vi "Create Map from Messages to Value Indexes.vi"(8 "error in":errorcluster, 9 "module reference":T3, 10 "1553 channel handles":T4[](array[typedef]) {"terminal status channels" format="%.0x"; "error count channel refs"."wrong sync" format="%.0x"; "error count channel refs"."word" format="%.0x"; "error count channel refs"."unconfigured frames" format="%.0x"; "error count channel refs"."parity" format="%.0x"; "error count channel refs"."monitor" format="%.0x"; "error count channel refs"."Manchester" format="%.0x"; "error count channel refs"."improper number of words" format="%.0x"; "error count channel refs"."general protocol" format="%.0x"; "messages"."Rx status handles" format="%.0x"; "messages"."Tx status handles" format="%.0x"; "messages"."timestamps" format="%.0x"; "messages"."parameters"."RxBC channel handle" format="%.0x"; "messages"."parameters"."RxRT channel handle" format="%.0x"; "messages"."parameters"."Tx channel handle" format="%.0x"}, 11 "1553 channels":T9[](array[typedef])) -> (0 "error out":errorcluster, 1 "Rx read info":T1[](array[typedef]), 2 "status lookup data":T2[](array[typedef]) {"terminal address" format="%.0x"; "remote terminal handle" format="%.0x"}, 3 "map from messages to value indexes":T17)   [LabVIEW 2020, in "AIM MIL-STD-1553 Engine.lvlib" / "Implementation.lvlib" / "Rx Execution Unit.lvclass"]
uses:
  Shared/Map of Messages to Value Indexes.ctl
  Shared/Message Map Key.ctl
  Implementation/Rx Execution Unit/Message Map Value.ctl
  Shared/Message Definition.ctl
  Shared/Message Type.ctl
  Shared/Terminal Endpoint.ctl
  Shared/Address.ctl
  Shared/Parameter Definition.ctl
  Shared/1553 Channel.ctl
  Shared/Major Frame Definition.ctl
  Shared/Minor Frame Definition.ctl
  Implementation/Execution Unit/1553 Channel Handles.ctl
  Implementation/Execution Unit/Message Handles.ctl
  Implementation/Execution Unit/Parameter Handles.ctl
  <vilib>/NI VeriStand/Custom Device API/Custom Device Item Ref.ctl
  Shared/Error Count Channel Refs.ctl
  Hardware API/Module Reference.ctl
  Implementation/Rx Execution Unit/Status Terminal Lookup Data.ctl
  Shared/Rx Read Info.ctl
  Implementation/Rx Execution Unit/Rx Execution Unit.lvclass
  Implementation/Address Based Execution Unit/Address Based Execution Unit.lvclass
  <vilib>/NI VeriStand/Custom Device API/Custom Device API.lvlib
  Implementation/Execution Unit/Execution Unit.lvclass
  Hardware API/AIM MIL-STD-1553 Hardware API.lvlib
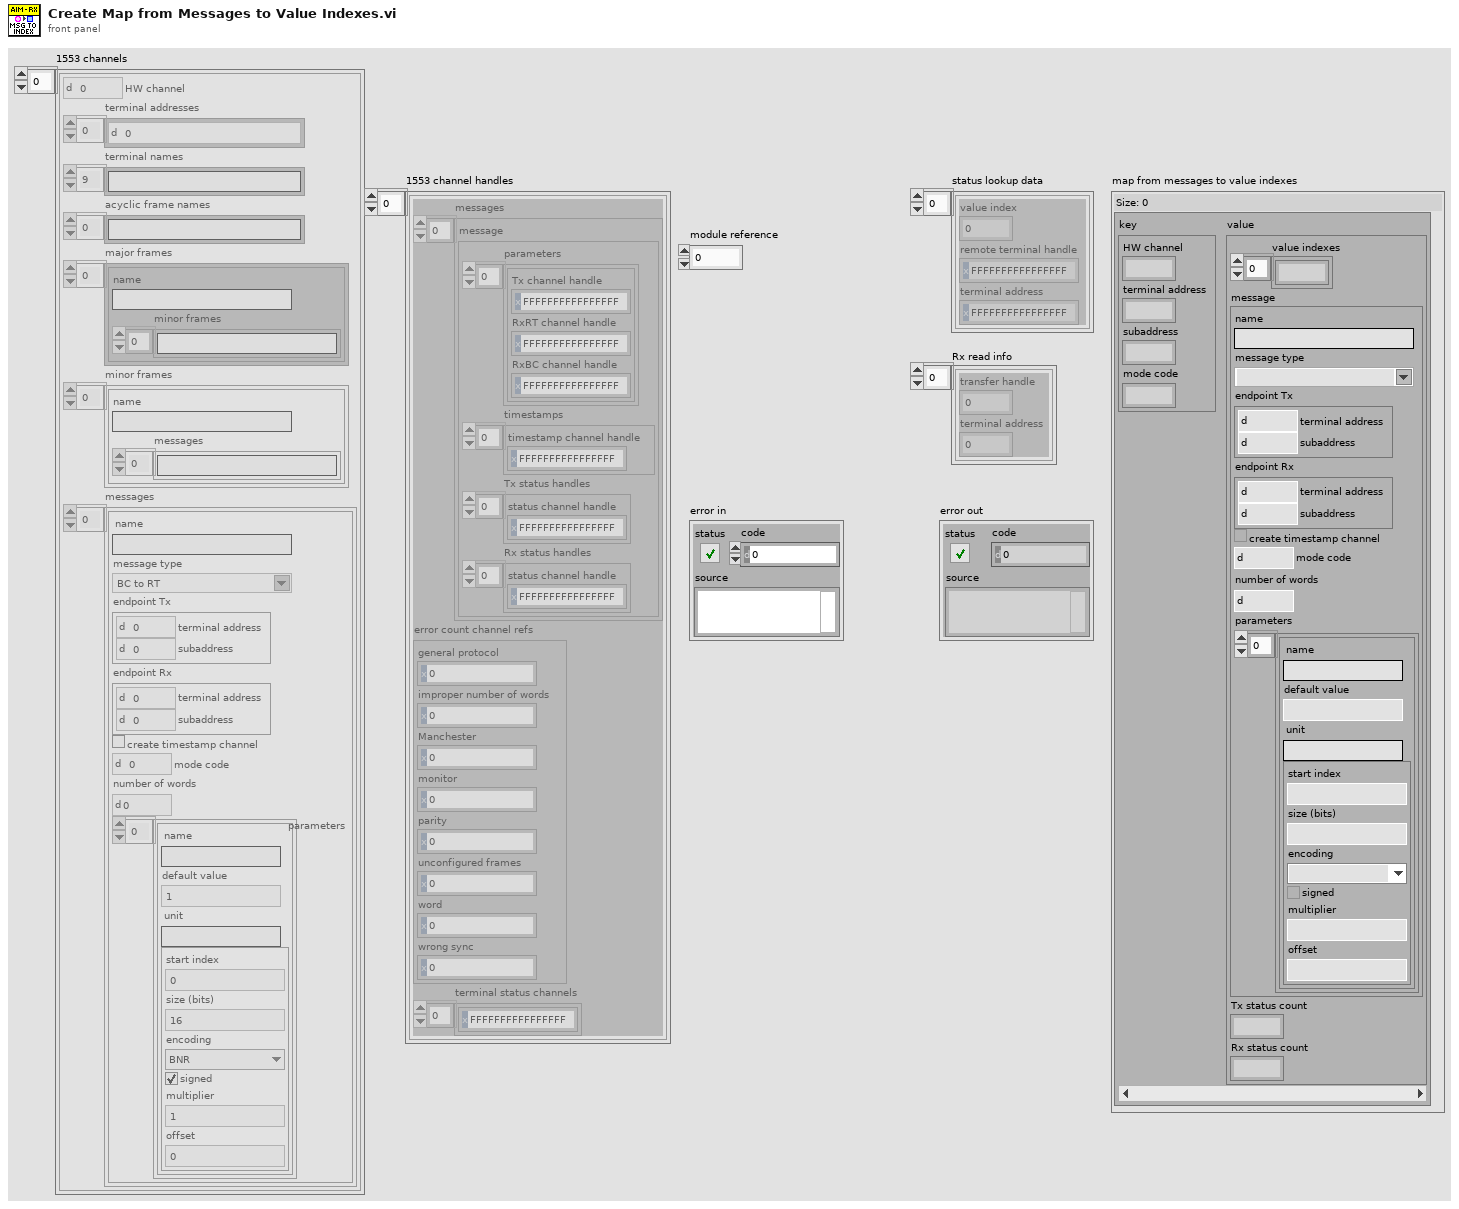
[diagram p1: front panel]
types:
  T1 = typedef "Rx Read Info.ctl" = cluster{"transfer handle":u64, "terminal address":u16}
  T2 = typedef "AIM MIL-STD-1553 Engine.lvlib/Implementation.lvlib/Rx Execution Unit.lvclass/Status Terminal Lookup Data.ctl" = cluster{"value index":i32, "remote terminal handle":u64, "terminal address":u64}
  T3 = typedef "AIM MIL-STD-1553 Hardware API.lvlib/Module Reference.ctl" = u32
  T4 = typedef "AIM MIL-STD-1553 Engine.lvlib/Implementation.lvlib/Execution Unit.lvclass/1553 Channel Handles.ctl" = cluster{"messages":T5[], "error count channel refs":T8, "terminal status channels":T7[]}
  T5 = typedef "AIM MIL-STD-1553 Engine.lvlib/Implementation.lvlib/Execution Unit.lvclass/Message Handles.ctl" = cluster{"parameters":T6[], "timestamps":T7[], "Tx status handles":T7[], "Rx status handles":T7[]}
  T6 = typedef "AIM MIL-STD-1553 Engine.lvlib/Implementation.lvlib/Execution Unit.lvclass/Parameter Handles.ctl" = cluster{"Tx channel handle":T7, "RxRT channel handle":T7, "RxBC channel handle":T7}
  T7 = typedef "Custom Device API.lvlib/Custom Device Item Ref.ctl" = u64
  T8 = typedef "Error Count Channel Refs.ctl" = cluster{"general protocol":T7, "improper number of words":T7, "Manchester":T7, "monitor":T7, "parity":T7, "unconfigured frames":T7, "word":T7, "wrong sync":T7}
  T9 = typedef "1553 Channel.ctl" = cluster{"HW channel":u16, "terminal addresses":T10[], "terminal names":string[], "acyclic frame names":string[], "major frames":T11[], "minor frames":T12[], "messages":T13[]}
  T10 = typedef "Address.ctl" = u16
  T11 = typedef "Major Frame Definition.ctl" = cluster{"name":string, "minor frames":string[]}
  T12 = typedef "Minor Frame Definition.ctl" = cluster{"name":string, "messages":string[]}
  T13 = typedef "Message Definition.ctl" = cluster{"name":string, "message type":T14, "endpoint Tx":T15, "endpoint Rx":T15, "create timestamp channel":bool, "mode code":u16, "number of words":u16, "parameters":cluster{"name":string, "default value":dbl, "unit":string, "parameter definition":T16}[]}
  T14 = typedef "Message Type.ctl" = string
  T15 = typedef "Terminal Endpoint.ctl" = cluster{"terminal address":T10, "subaddress":T10}
  T16 = typedef "Parameter Definition.ctl" = cluster{"start index":i32, "size (bits)":i32, "encoding":enum16{"BNR", "BCD", "Discrete"}, "signed":bool, "multiplier":dbl, "offset":dbl}
  T17 = typedef "Map of Messages to Value Indexes.ctl" = map{T18, T19}
  T18 = typedef "Message Map Key.ctl" = cluster{"HW channel":u16, "terminal address":u16, "subaddress":u16, "mode code":u16}
  T19 = typedef "AIM MIL-STD-1553 Engine.lvlib/Implementation.lvlib/Rx Execution Unit.lvclass/Message Map Value.ctl" = cluster{"value indexes":i32[], "message":T13, "Tx status count":i32, "Rx status count":i32}
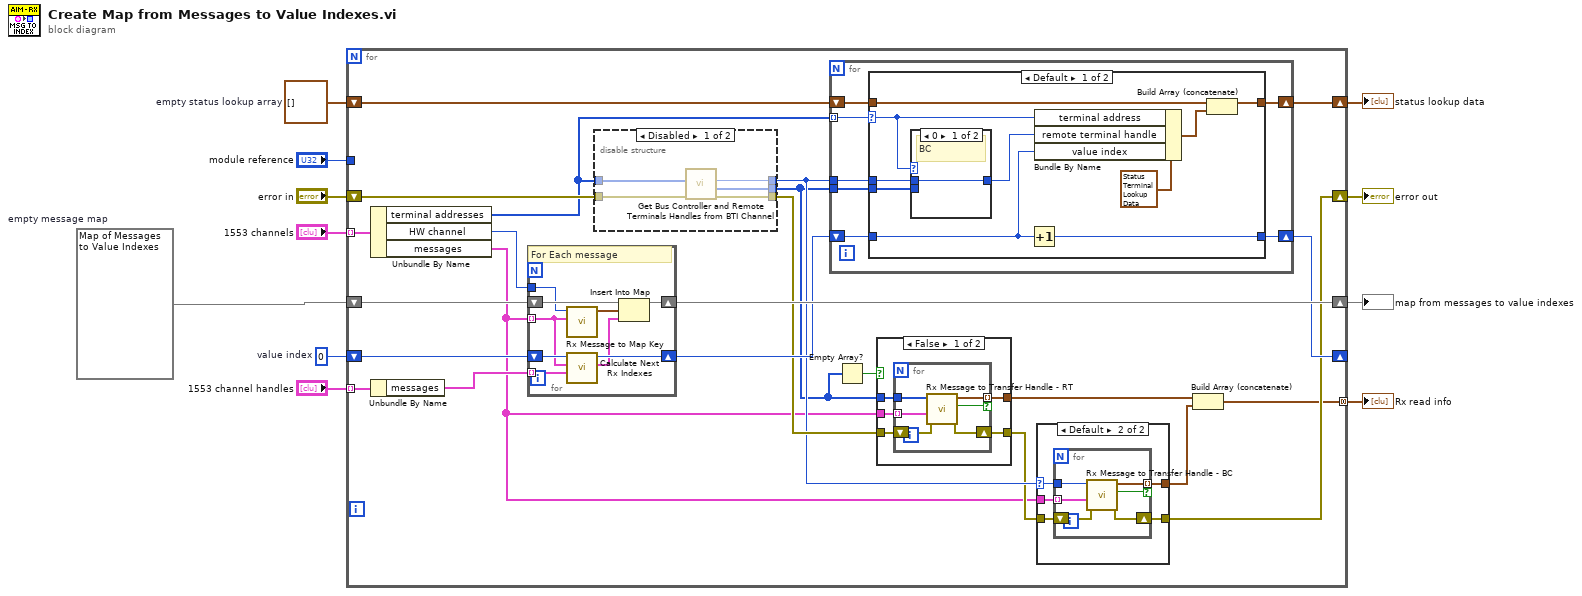
[diagram p0: block diagram]
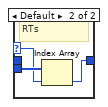
[diagram p5: hidden frame]
diagram:
  w3 = T2[] []  # empty status lookup array
  w9 = 0  # value index
  w11 = T17 {}  # empty message map
  n1 = for {
    tunnel: "1553 channels" -> [w30] mode=indexing
    shift-right: [w32] -> w7
    shift-left: w11 -> [w34]
    shift-right: [w25] -> _
    shift-left: w9 -> [w33]
    tunnel: "1553 channel handles" -> [w28] mode=indexing
    tunnel: "module reference" -> [_]
    shift-right: [w17] -> w5
    shift-left: "error in" -> [w24]
    shift-right: [w27] -> w2
    shift-left: w3 -> [w29]
    tunnel: [w12] -> w1 mode=concatenating
    n2 = Unbundle By Name(w30) -> ("terminal addresses"=w22:T10[], "HW channel"=w23:u16, "messages"=w13:T13[])
    n3 = Unbundle By Name(w28) -> ("messages"=w31:T5[])
    n4 = for {
      tunnel: w23 -> [w71]
      tunnel: w13 -> [w67] mode=indexing
      shift-right: [w73] -> w32
      shift-left: w34 -> [w72]
      shift-right: [w70] -> w26
      shift-left: w33 -> [w69]
      tunnel: w31 -> [w65] mode=indexing
      # "For Each message"
      n5 = call "Rx Message to Map Key.vi"("message"=w67, "HW channel"=w71) -> ("message map key"=w68:T18)  [unwired: 9 in]
      n6 = call "Calculate Next Rx Indexes.vi"("message handles"=w65, "message"=w67, "index"=w69) -> ("message map value"=w66:T19, "next index"=w70:i32)  [unwired: 7 in]
      n7 = Insert Into Map(map in=w72, key=w68, value=w66) -> (map out=w73:T17)  [unwired: 2 out]
    }
    n8 = disable-structure shown="Disabled" {
      disable-tunnel: w24 -> [w39 w40]
      disable-tunnel: w22 -> [w38 _]
      disable-tunnel: [w37 w40] -> w21
      disable-tunnel: [w36 _] -> w19
      disable-tunnel: [w35 _] -> w14
      frame Disabled {
        n9 = call "Get Bus Controller and Remote Terminals Handles from BTI Channel.vi"("error in"=w39, "terminal addresses"=w38) -> ("error out"=w37:errorcluster, "remote terminal handles out"=w35:u64[], "bus controller handle out"=w36:u64)  [unwired: 6 in, 1 out]
      }
      frame Enabled {
        # "#AIM get BC and RT handles"
      }
    }
    n10 = for {
      tunnel: w22 -> [w74] mode=indexing
      shift-right: [w80] -> w27
      shift-left: w29 -> [w79]
      tunnel: w14 -> [w78]
      tunnel: w19 -> [w77]
      shift-right: [w75] -> w25
      shift-left: w26 -> [w76]
      n11 = case shown="Default" w74 {
        selector: w74 -> [w82 _]
        tunnel: [w84 w96] -> w80
        tunnel: w79 -> [w85 w96]
        tunnel: w78 -> [w90 _]
        tunnel: w77 -> [w89 _]
        tunnel: w76 -> [w81 w95]
        tunnel: [w86 w95] -> w75
        frame Default {
          n12 = case shown="0" w82 {
            selector: w82 -> [_ w93]
            tunnel: w90 -> [_ w94]
            tunnel: w89 -> [w91 _]
            tunnel: [w91 w92] -> w87
            frame 0 {
              # "BC"
            }
            frame Default {
              # "RTs"
              n13 = Index Array(array=w94, index=w93) -> (element=w92:u64)
            }
          }
          n14 = Increment(x=w81) -> (x+1=w86:i32)
          n15 = Bundle By Name(cluster=T2 {"value index"=0, "remote terminal handle"=18446744073709551615, "terminal address"=18446744073709551615} ("value"), "terminal address"=w82, "remote terminal handle"=w87, "value index"=w81) -> (w83:T2)
          n16 = Build Array (concatenate)(w85, w83) -> (w84:T2[])
        }
        frame 31 {
        }
      }
    }
    n17 = Empty Array?(array=w14) -> (empty?=w15:bool)
    n18 = case shown="False" w15 {
      tunnel: w13 -> [w45 _]
      tunnel: w14 -> [w44 _]
      tunnel: w21 -> [w43 w52]
      tunnel: [w42 w52] -> w18
      tunnel: [w41 _] -> w20
      frame False {
        n19 = for {
          tunnel: w45 -> [w51] mode=indexing
          tunnel: w44 -> [w46]
          shift-right: [w49] -> w42
          shift-left: w43 -> [w50]
          tunnel: [w48] -> w41 mode=indexing if=w47
          n20 = call "Rx Message to Transfer Handle - RT.vi"("error in"=w50, "message"=w51, "remote terminal handles"=w46) -> ("error out"=w49:errorcluster, "valid?"=w47:bool, "Rx read info"=w48:T1)  [unwired: 6 in]
        }
      }
      frame True {
      }
    }
    n21 = case shown="Default" w19 {
      selector: w19 -> [_ w54]
      tunnel: w13 -> [_ w58]
      tunnel: w18 -> [w53 w57]
      tunnel: [w53 w56] -> w17
      tunnel: [_ w55] -> w16
      frame 0 {
      }
      frame Default {
        n22 = for {
          tunnel: w58 -> [w64] mode=indexing
          shift-right: [w62] -> w56
          shift-left: w57 -> [w63]
          tunnel: [w61] -> w55 mode=indexing if=w60
          tunnel: w54 -> [w59]
          n23 = call "Rx Message to Transfer Handle - BC.vi"("error in"=w63, "message"=w64, "bus controller handle"=w59) -> ("error out"=w62:errorcluster, "valid?"=w60:bool, "Rx read info"=w61:T1)  [unwired: 6 in]
        }
      }
    }
    n24 = Build Array (concatenate)(w20, w16) -> (w12:T1[])
  }
  "map from messages to value indexes" <- w7
  "error out" <- w5
  "status lookup data" <- w2
  "Rx read info" <- w1
